vi "GeraSinalComposto.vi"(0 "params":variant, 2 "Tx Aquisicao":dbl, 4 "estadoIn":variant) -> (15 "sinal":waveform(dbl), 18 "estadoOut":variant)   [LabVIEW 2017]
uses:
  Typedefs/Tipo_ParamsComposto.ctl
  Typedefs/Tipo_ComponenteSinalComposto.ctl
  <vilib>/Analysis/NI_AALBase.lvlib
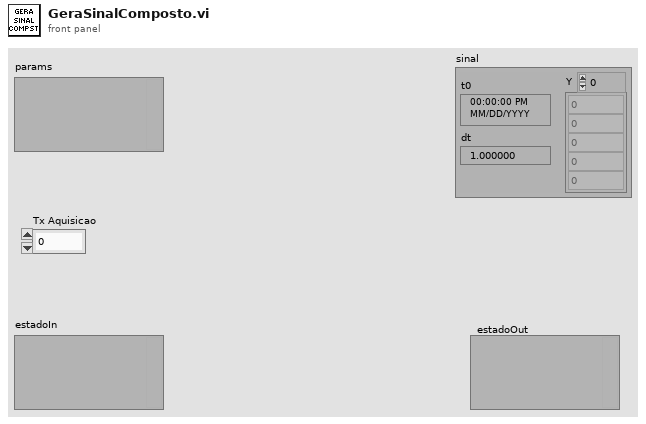
[diagram p1: front panel]
types:
  T1 = typedef "Tipo_ParamsComposto.ctl" = cluster{"Componentes":T2[], "Ruído":dbl}
  T2 = typedef "Tipo_ComponenteSinalComposto.ctl" = cluster{"Amplit.: ":dbl, "Freq. (Hz): ":dbl, "Fase (º):":dbl}
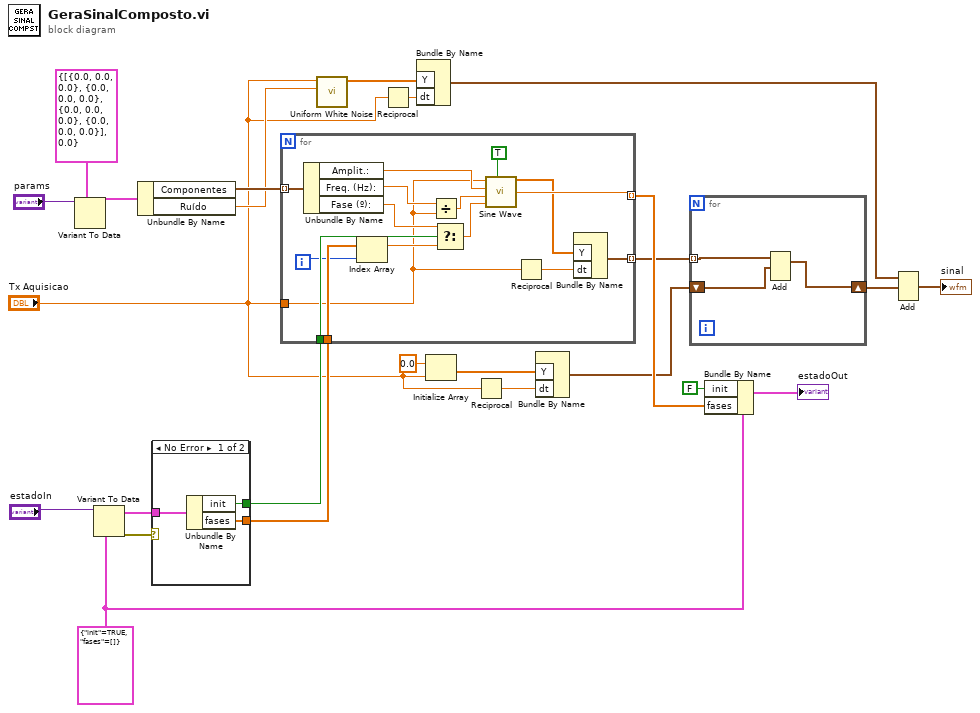
[diagram p0: block diagram]
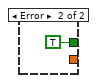
[diagram p2: hidden frame]
diagram:
  w16 = cluster{"init":bool, "fases":dbl[]} {"init"=TRUE, "fases"=[]}
  n1 = Variant To Data(type=T1 {"Componentes"=[{"Amplit.: "=0.0, "Freq. (Hz): "=0.0, "Fase (º):"=0.0}, {"Amplit.: "=0.0, "Freq. (Hz): "=0.0, "Fase (º):"=0.0}, {"Amplit.: "=0.0, "Freq. (Hz): "=0.0, "Fase (º):"=0.0}, {"Amplit.: "=0.0, "Freq. (Hz): "=0.0, "Fase (º):"=0.0}], "Ruído"=0.0} ("Cluster"), Variant="params") -> (data=w23:T1)  [unwired: 1 in, 1 out]
  n2 = Variant To Data(type=w16, Variant="estadoIn") -> (data=w20:cluster{"init":bool, "fases":dbl[]}, error out=w17:errorcluster)  [unwired: 1 in]
  n3 = Unbundle By Name(w23) -> ("Componentes"=w22:T2[], "Ruído"=w9:dbl)
  n4 = case shown="No Error" w17 {
    tunnel: w20 -> [w28 _]
    tunnel: [w27 TRUE ("init")] -> w19
    tunnel: [w26 _] -> w18
    frame No Error {
      n5 = Unbundle By Name(w28) -> ("init"=w27:bool, "fases"=w26:dbl[])
    }
    frame Error {
    }
  }
  n6 = for {
    tunnel: w22 -> [w39] mode=indexing
    tunnel: w19 -> [w44]
    tunnel: w18 -> [w41]
    tunnel: [w40] -> w13 mode=indexing
    tunnel: "Tx Aquisicao" -> [w31]
    tunnel: [w30] -> w12 mode=indexing
    i -> [w34]
    n7 = Unbundle By Name(w39) -> ("Amplit.:"=w38:dbl, "Freq. (Hz):"=w37:dbl, "Fase (º):"=w36:dbl)
    n8 = Index Array(array=w41, index=w34) -> (element=w35:dbl)
    n9 = Divide(x=w37, y=w31) -> (x/y=w45:dbl)
    n10 = Select(t=w36, s=w44, f=w35) -> (s? t:f=w43:dbl)
    n11 = call <vilib>:"Sine Wave.vi"("samples"=w31, "amplitude"=w38, "frequency"=w45, "phase in"=w43, "reset phase"=TRUE) -> ("sine wave"=w32:dbl[], "phase out"=w40:dbl)  [unwired: 1 out]
    n12 = Reciprocal(x=w31) -> (1/x=w33:dbl)
    n13 = Bundle By Name("Y"=w32, "dt"=w33) -> (w30:waveform(dbl))  [unwired: 1 in]
  }
  n14 = call <vilib>:"Uniform White Noise.vi"("amplitude"=w9, "samples"="Tx Aquisicao") -> ("uniform white noise"=w8:dbl[])  [unwired: 8 in, 1 out]
  n15 = Reciprocal(x="Tx Aquisicao") -> (1/x=w7:dbl)
  n16 = Bundle By Name("Y"=w8, "dt"=w7) -> (w6:waveform(dbl))  [unwired: 1 in]
  n17 = Initialize Array(0.0 ("element"), "Tx Aquisicao") -> (w4:dbl[])
  n18 = Reciprocal(x="Tx Aquisicao") -> (1/x=w2:dbl)
  n19 = Bundle By Name("Y"=w4, "dt"=w2) -> (w1:waveform(dbl))  [unwired: 1 in]
  n20 = for {
    tunnel: w12 -> [w48] mode=indexing
    shift-right: [w46] -> w11
    shift-left: w1 -> [w47]
    n21 = Add(1:w47, 2:w48) -> (0:w46:waveform(dbl))  [unwired: 1 in, 1 out]
  }
  n22 = Bundle By Name(cluster=w16, "init"=FALSE, "fases"=w13) -> (→"estadoOut":cluster{"init":bool, "fases":dbl[]})
  n23 = Add(1:w11, 2:w6) -> (0:→"sinal":waveform(dbl))  [unwired: 1 in, 1 out]
